vi "ReadSerialAndAnalysis_MoreCodeNeeded.vi"() -> ()   [LabVIEW 2023]
doc: "This example performs writes and reads on a serial port, as directed by the user. You can press the Write and Read buttons, and change the Read Count, while the example is running.\n\nThe parameters set for the serial port must match the parameters of the connected instrument or device. In this example, the Read Count parameter specifies the number of bytes that the serial port reads. If there were more bytes at the port than the specified number, those bytes would not be read. If there were less bytes at the port than the specified number, you would receive a timeout error.\n\nThis example expands upon the flow control options for XON and XOFF, allowing the user to choose those control characters. Also, the user can enable or disable a termination character. Some devices require a termination character in order to identify the end of command strings. Some devices send a termination character to signify the end of data to be read. This example shows how you can end the Read operation once a termination character is detected in the buffer and/or append a termination character at the end of the Write data."
uses:
  includes/enumFGVstringBuffer.ctl
panel:
  in  "Serial resource":refnum<visa-resource-name>="COM1"
  in  "Stop":bool
  out "One data line":string
  in  "data length to process":i32=200
  out "Time data":waveform(dbl)[](graph)
  out "Mean (all channels)":dbl[](array[numeric])
  out "Std (all channels)":dbl[](array[numeric])
  out "Variancce (all channels)":dbl[](array[numeric])
  out "PSD":cluster{"f0":dbl, "df":dbl, "magnitude":dbl[]}[](graph)
  out "Histogram Graph":T1(graph)
  out "Skewness (all channels)":dbl[](array[numeric])
  out "Kurtosis (all channels)":dbl[](array[numeric])
  out "Median Noise (all channels)":dbl[](array[numeric])
  out "Raw data":dbl[][](graph)
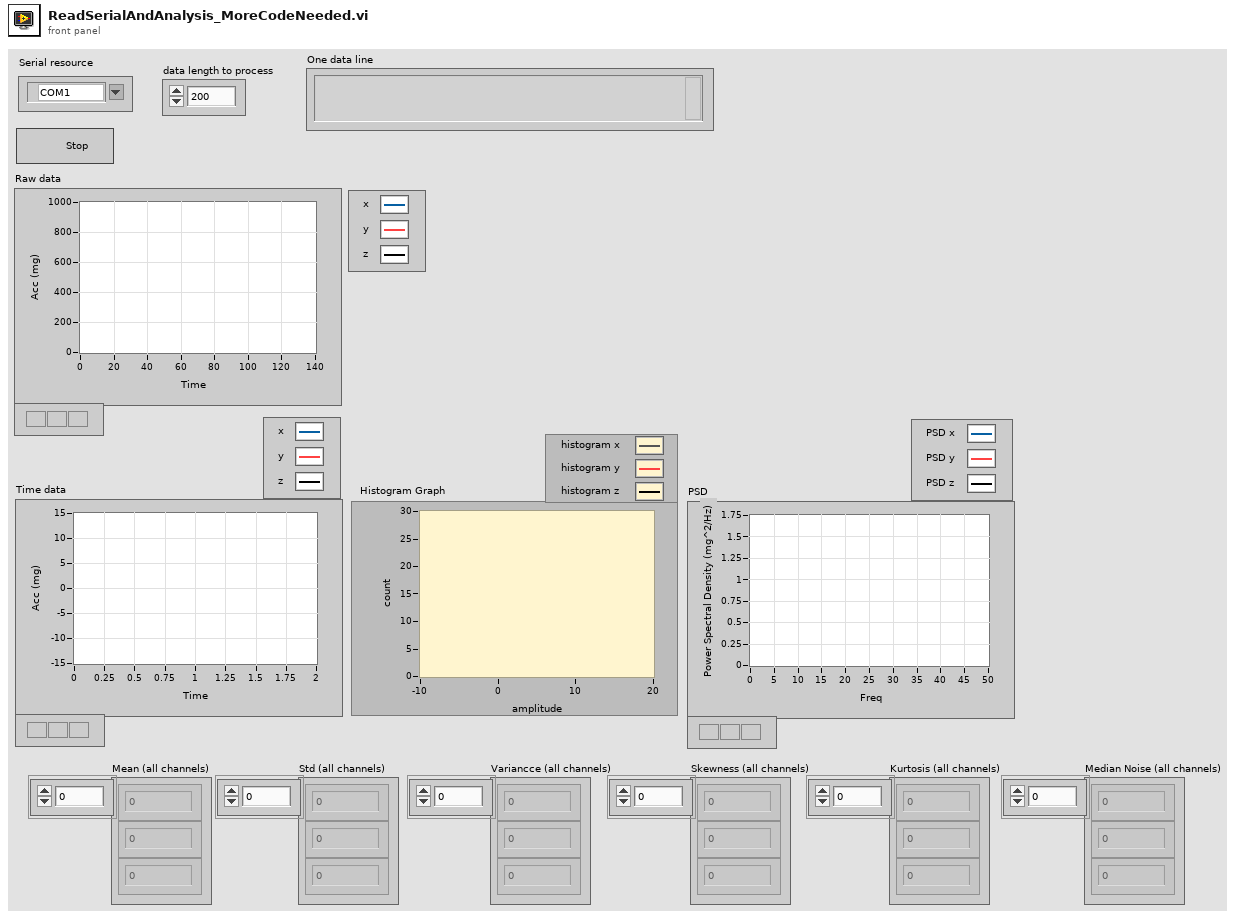
[diagram p1: front panel]
types:
  T1 = cluster{"X Values":dbl[], "Histogram: h(x)":i32[]}[]
  T2 = typedef "enumFGVstringBuffer.ctl" = enum16{"Init", "Write", "Read"}
  T3 = cluster{"Mean (all channels)":dbl[], "Std (all channels)":dbl[], "Variancce (all channels)":dbl[], "Skewness (all channels)":dbl[], "Kurtosis (all channels)":dbl[], "Median Noise (all channels)":dbl[]}
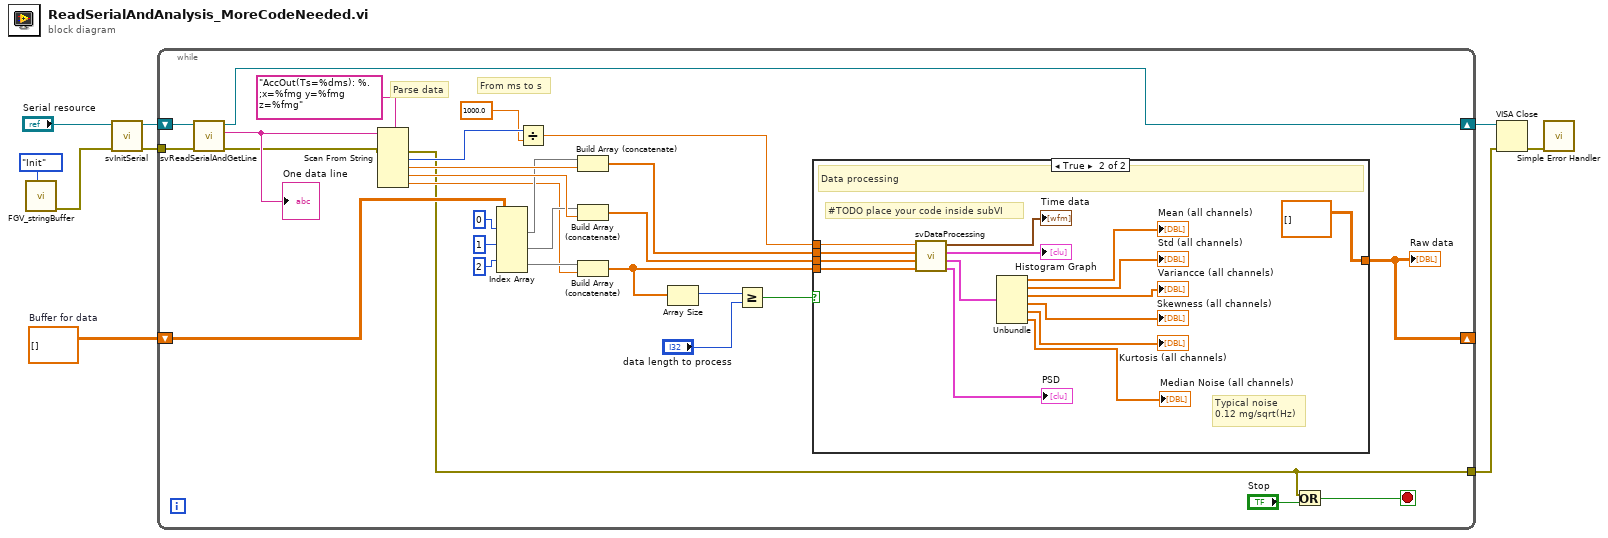
[diagram p0: block diagram]
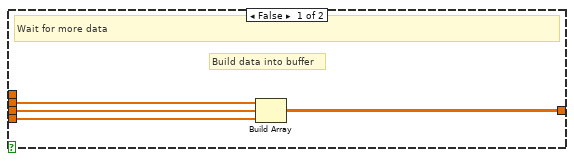
[diagram p2: hidden frame]
diagram:
  w4 = dbl[][] []  # Buffer for data
  n1 = call "FGV_stringBuffer.vi"("Enum"=enumFGVstringBuffer."Init") -> ("error out"=w2:errorcluster)  [unwired: 9 in, 1 out]
  n2 = call "svInitSerial.vi"("error in"=w2, "VISA Refnum in"="Serial resource") -> ("error out"=w6:errorcluster, "VISA Refnum out"=w5:refnum<visa-resource-name>)  [unwired: 8 in]
  n3 = while {
    shift-right: [w19] -> w7
    shift-left: w5 -> [w38]
    tunnel: w6 -> [w37]
    shift-right: [w11] -> _
    shift-left: w4 -> [w33]
    tunnel: [w10] -> w1
    stop <- w36 stop-if-true
    # "From ms to s"
    # "Parse data"
    # "Serial Read Loop"
    n4 = call "svReadSerialAndGetLine.vi"("error in (no error)"=w37, "VISA Refnum in"=w38) -> ("error out"=w20:errorcluster, "One data line"=w21:string, "VISA Refnum out"=w19:refnum<visa-resource-name>)  [unwired: 7 in]
    "One data line" <- w21
    n5 = Scan From String(format string="AccOut(Ts=%dms): %.;x=%fmg y=%fmg z=%fmg", input string=w21, error in=w20) -> (error out=w10:errorcluster, output 1=w34:i32, output 2=w30:dbl, output 3=w29:dbl, output 4=w22:dbl)  [unwired: 5 in, 2 out]
    n6 = Index Array(array=w33, index (row) #1=0 ("index (row)"), index (row) #2=1 ("index (row)"), index (row) #3=2 ("index (row)")) -> (element #1=w26:dbl[], element #2=w25:dbl[], element #3=w23:dbl[])  [unwired: 3 in]
    n7 = Divide(x=w34, y=1000.0) -> (x/y=w16:dbl)
    n8 = Build Array (concatenate)(w26, w30) -> (w13:dbl[])
    n9 = Build Array (concatenate)(w25, w29) -> (w14:dbl[])
    n10 = Build Array (concatenate)(w23, w22) -> (w15:dbl[])
    n11 = Array Size(array=w15) -> (size(s)=w18:i32)
    n12 = Greater Or Equal?(x=w18, y="data length to process") -> (x >= y?=w17:bool)
    n13 = case shown="True" w17 {
      tunnel: w16 -> [_ w56]
      tunnel: w15 -> [w40 w53]
      tunnel: w14 -> [w41 w54]
      tunnel: w13 -> [w42 w55]
      tunnel: [w39 dbl[][] []] -> w11
      frame False {
        # "Build data into buffer"
        # "Wait for more data"
        n14 = Build Array(w42, w41, w40) -> (w39:dbl[][])
      }
      frame True {
        # "#TODO place your code inside subVI"
        # "Typical noise\n0.12 mg/sqrt(Hz)"
        # "Data processing"
        n15 = call "svDataProcessing.vi"("Z axis"=w53, "Y axis"=w54, "X axis"=w55, "dt"=w56) -> ("PSD"=→"PSD":cluster{"f0":dbl, "df":dbl, "magnitude":dbl[]}[], "statistical data"=w50:T3, "Histogram Graph"=→"Histogram Graph":T1, "Time data"=→"Time data":waveform(dbl)[])  [unwired: 2 in]
        n16 = Unbundle(w50) -> ("Mean (all channels)"=→"Mean (all channels)":dbl[], "Std (all channels)"=→"Std (all channels)":dbl[], "Variancce (all channels)"=→"Variancce (all channels)":dbl[], "Skewness (all channels)"=→"Skewness (all channels)":dbl[], "Kurtosis (all channels)"=→"Kurtosis (all channels)":dbl[], "Median Noise (all channels)"=→"Median Noise (all channels)":dbl[])
      }
    }
    "Raw data" <- w11
    n17 = Or(x=w10, y="Stop") -> (x .or. y?=w36:bool)
  }
  n18 = VISA Close(VISA resource name=w7, error in (no error)=w1) -> (error out=w8:errorcluster)
  n19 = call <vilib>:"Simple Error Handler.vi"("error in (no error)"=w8) -> ()  [unwired: 1 in, 8 out]
